vi "MPU6050 Tester.vi"() -> ()   [LabVIEW 2020]
uses:
  Typedefs/LED mode.ctl
  Typedefs/Front Panel Object References.ctl
  Typedefs/GUI Command Cluster.ctl
  Typedefs/GUI Commands.ctl
  Typedefs/SDCP - Standard Message Frame Parameters - FGV - commands.ctl
  Typedefs/SDCP - Serial Port Control - Commands.ctl
  Global Variables/Application Stop.vi
panel:
  in  "Exit Application":bool
  in  "Switch":bool
  in  "Anti clockwise":bool
  in  "Clockwise":bool
  out "Z vibration detected":bool
  out "Y vibration detected":bool
  out "X vibration detected":bool
  out "Z tilt detected":bool
  out "Y tilt detected":bool
  out "X tilt detected":bool
  in  "Save config":bool
  out "Yaw (degrees)":dbl
  out "Pitch (degrees)":dbl
  out "Roll (degrees)":dbl
  in  "Calibrate IMU":bool
  out "IMU orientation":refnum<vi>(3d-picture)
  in  "Serial Port Connect":bool
  in  "Write config":bool
  in  "Read config":bool
  out "Z gyroscope (mDPS)":u16
  out "Y gyroscope (mDPS)":u16
  out "X gyroscope  (mDPS)":u16
  out "Z accelerometer (mG)":u16
  out "Y accelerometer (mG)":u16
  out "X accelerometer (mG)":u16
  out "Z gyroscope raw":u16
  out "Y gyroscope raw":u16
  out "X gyroscope raw":u16
  out "Z accelerometer raw":u16
  out "Y accelerometer raw":u16
  out "X accelerometer raw":u16
  in  "Z LED mode":T1
  in  "Y LED mode":T1
  in  "X LED mode":T1
  in  "Z vib threshold":dbl
  in  "Y vib threshold":dbl
  in  "X vib threshold":dbl
  in  "Z tilt threshold":dbl
  in  "Y tilt threshold":dbl
  in  "X tilt threshold":dbl
  in  "Yaw coefficient":dbl
  in  "Pitch coefficient":dbl
  in  "Roll coefficient":dbl
  in  "Calibration Axis":T2(ring)
  in  "Calibration Points":u8
  in  "Calibration interval (ms)":u8
  in  "Gyroscope full scale value":enum16{"250DPS", "500DPS", "1000DPS", "2000DPS"}(ring)
  in  "Accelerometer full scale value":enum16{"2G", "4G", "8G", "16G"}(ring)
  in  "Baud rate":u32=9600
  in  "COM Port":refnum<visa-resource-name>
  # "IMU Configurations"
  # "Serial Port Configurations"
  # "IMU Raw measurements"
  # "Complementary Filter Configurations"
  # "Tilt Detection Configurations"
  # "IMU Processed measurements"
  # "Vibration Detection Configurations"
  # "LED Configurations"
  # "Screen control"
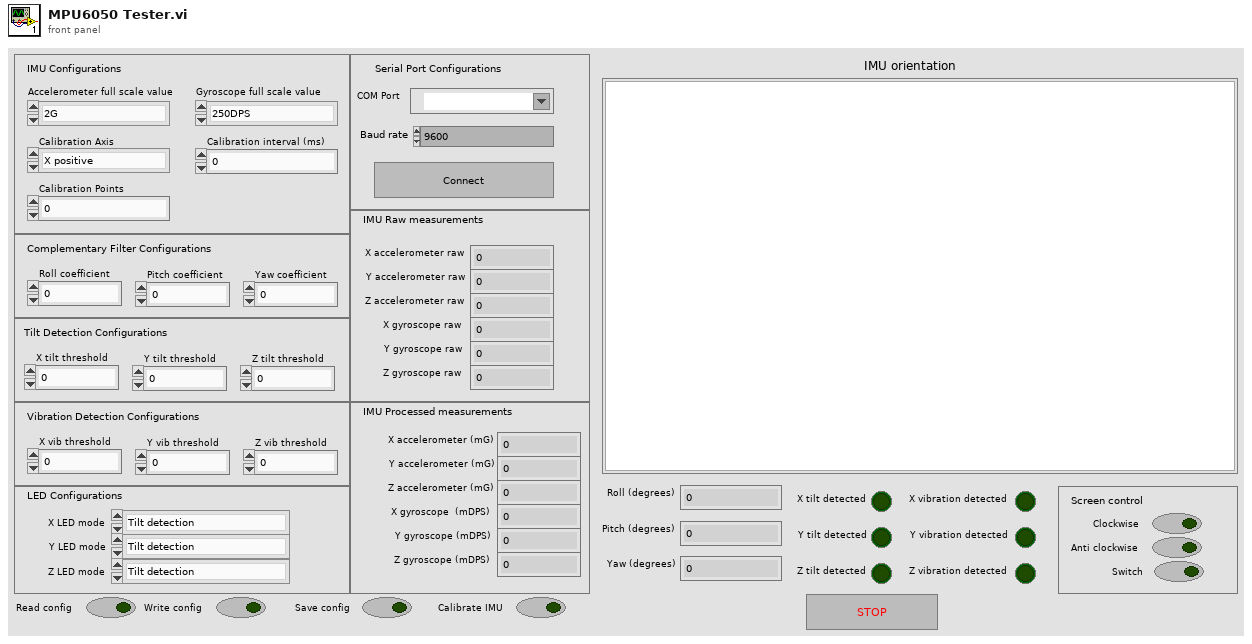
[diagram p1: front panel]
types:
  T1 = typedef "LED mode.ctl" = enum16{"Tilt detection", "Vibration detection", "Accelerometer magnitude", "Gyroscope magnitude", "GPIO test", "PWM test"}
  T2 = enum16{"X positive", "X neagtive", "Y positive", "Y negative", "Z positive", "Z negative"}
  T3 = typedef "SDCP - Standard Message Frame Parameters - FGV - commands.ctl" = enum16{"Write descriptors", "Read descriptors", "Read values", "Load parameters from file", "Write values", "Read all descriptors"}
  T4 = typedef "GUI Command Cluster.ctl" = cluster{"Command":T5, "Data":variant}
  T5 = typedef "GUI Commands.ctl" = enum16{"Serial Port Connect", "Serial Port Disconnect", "Read config", "Write config", "Save config", "Calibrate", "RENC CLK", "RENC ACLK", "RENC SW", "Exit Application"}
  T6 = typedef "Front Panel Object References.ctl" = cluster{"Switch":refnum<vi>, "Anti clockwise":refnum<vi>, "Clockwise":refnum<vi>, "Save config":refnum<vi>, "Calibrate IMU":refnum<vi>, "Serial Port Connect":refnum<vi>, "Write config":refnum<vi>, "Read config":refnum<vi>, "Z LED mode":refnum<vi>, "Y LED mode":refnum<vi>, "X LED mode":refnum<vi>, "Z vib threshold":refnum<vi>, "Y vib threshold":refnum<vi>, "X vib threshold":refnum<vi>, "Z tilt threshold":refnum<vi>, "Y tilt threshold":refnum<vi>, "X tilt threshold":refnum<vi>, "Yaw coefficient":refnum<vi>, "Pitch coefficient":refnum<vi>, "Roll coefficient":refnum<vi>, "Calibration Axis":refnum<vi>, "Calibration Points":refnum<vi>, "Calibration interval (ms)":refnum<vi>, "Gyroscope full scale value":refnum<vi>, "Accelerometer full scale value":refnum<vi>, "Baud rate":refnum<vi>, "COM Port":refnum<vi>, "Z vibration detected":refnum<vi>, "Y vibration detected":refnum<vi>, "X vibration detected":refnum<vi>, "Z tilt detected":refnum<vi>, "Y tilt detected":refnum<vi>, "X tilt detected":refnum<vi>, "Yaw (degrees)":refnum<vi>, "Pitch (degrees)":refnum<vi>, "Roll (degrees)":refnum<vi>, "IMU orientation":refnum<vi>, "Z gyroscope raw (mDPS)":refnum<vi>, "Y gyroscope (mDPS)":refnum<vi>, "X gyroscope raw (mDPS)":refnum<vi>, "Z accelerometer raw (mG)":refnum<vi>, "Y accelerometer raw (mG)":refnum<vi>, "X accelerometer (mG)":refnum<vi>, "Z gyroscope raw":refnum<vi>, "Y gyroscope raw":refnum<vi>, "X gyroscope raw":refnum<vi>, "Z accelerometer raw":refnum<vi>, "Y accelerometer raw":refnum<vi>, "X accelerometer raw":refnum<vi>}
  T7 = typedef "SDCP - SMF parameter descriptors.ctl" = cluster{"Frame name":string, "Frame ID":i32, "Data type":string, "Start Position":i32, "Length":i32, "Factor":dbl, "Offset":dbl, "Parameter name":string, "Value":string}
  T8 = typedef "SDCP - Serial Port Control - Commands.ctl" = enum16{"Open", "Read", "Write", "Get instance", "Close"}
  T9 = enum8{"Enabled", "Disabled", "Disabled and Grayed Out"}
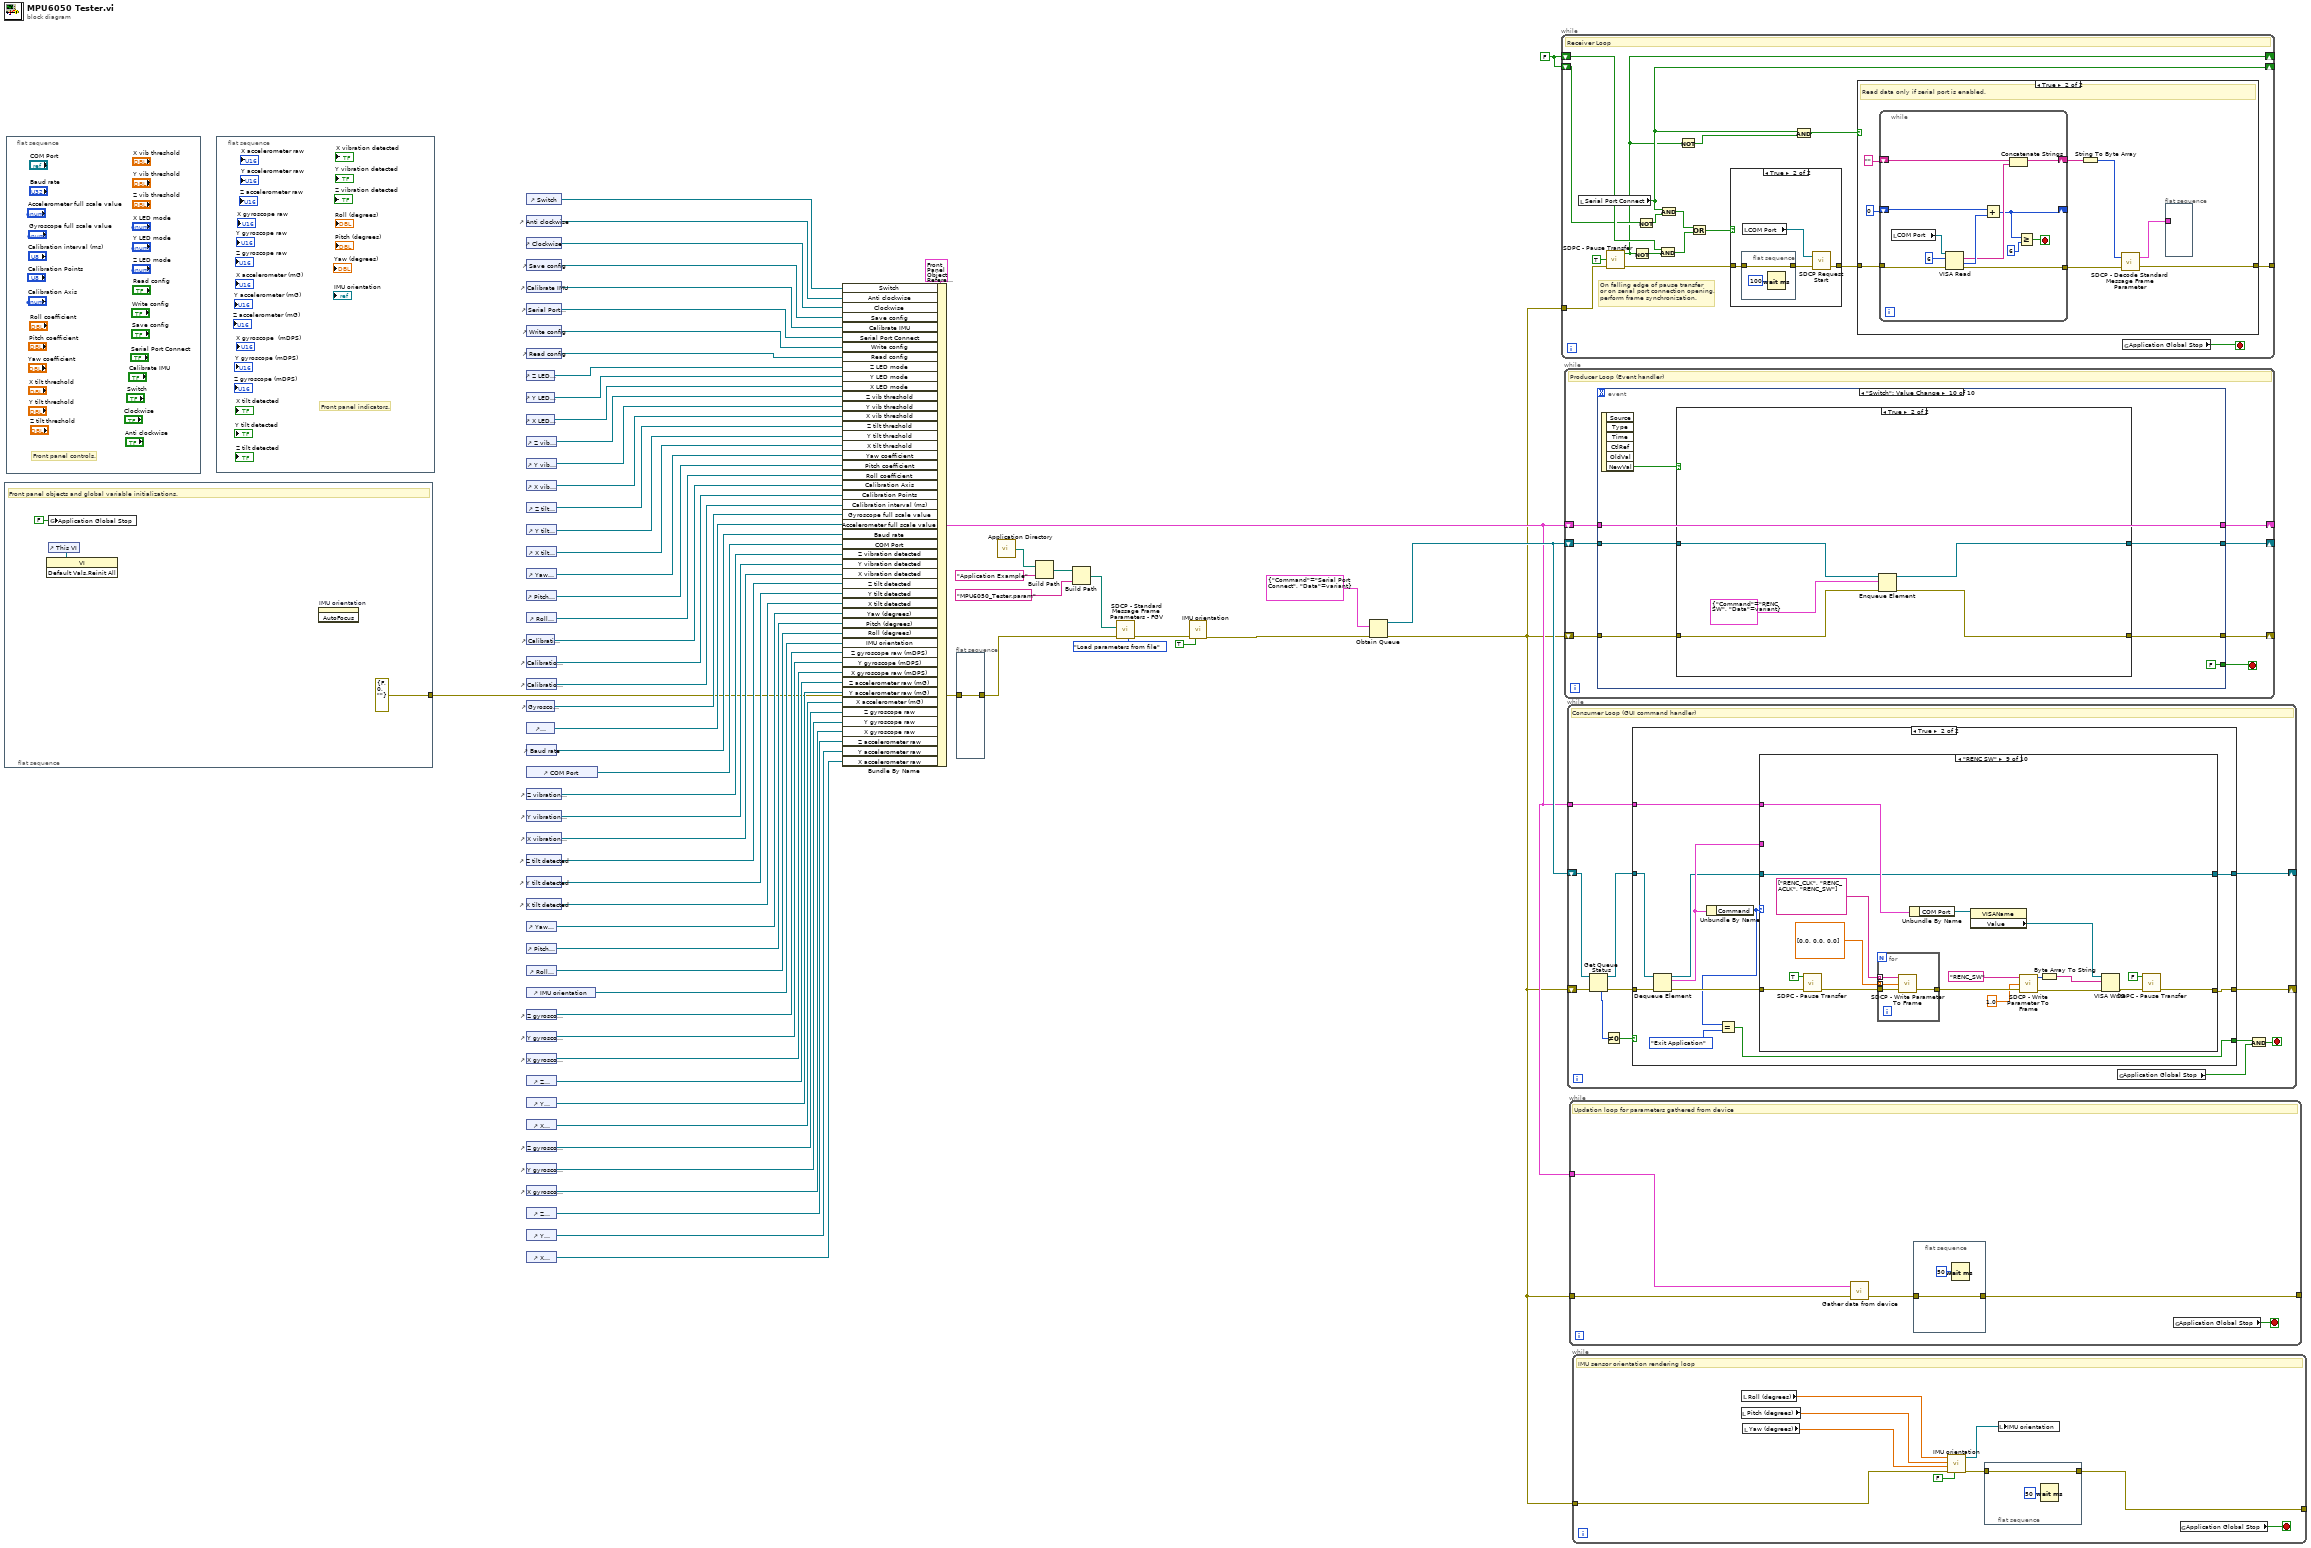
[diagram p0: block diagram]
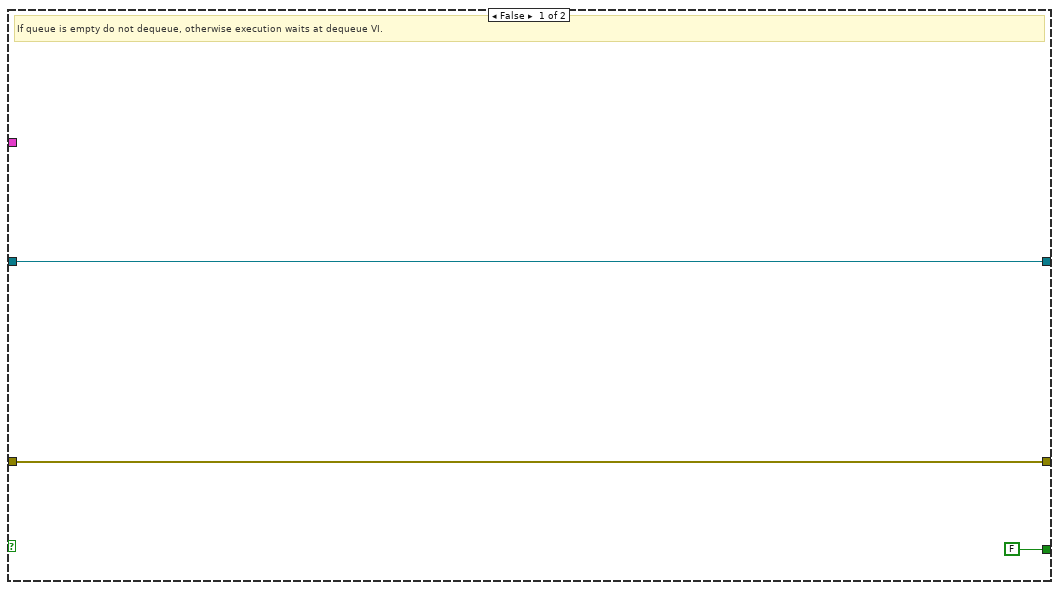
[diagram p4: hidden frame]
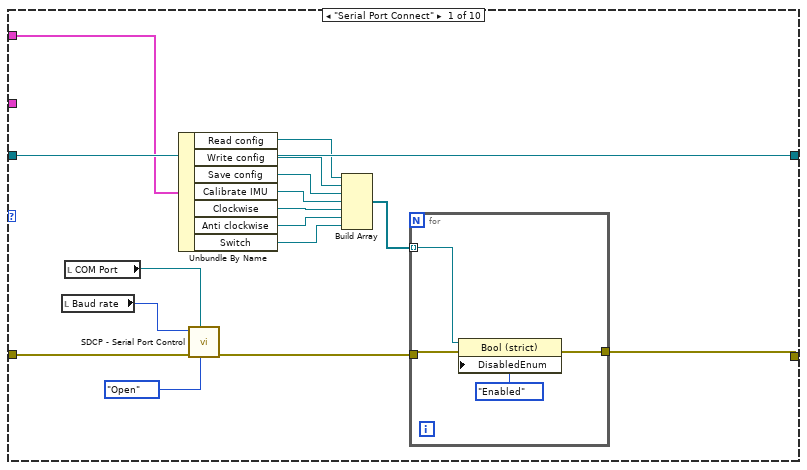
[diagram p5: hidden frame]
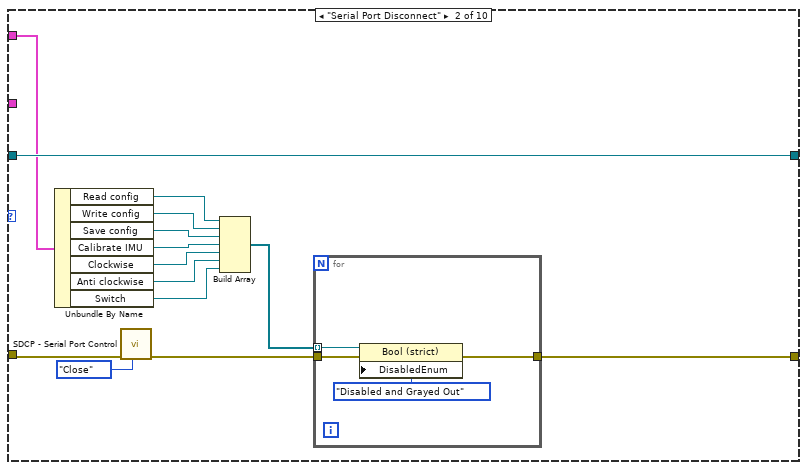
[diagram p6: hidden frame]
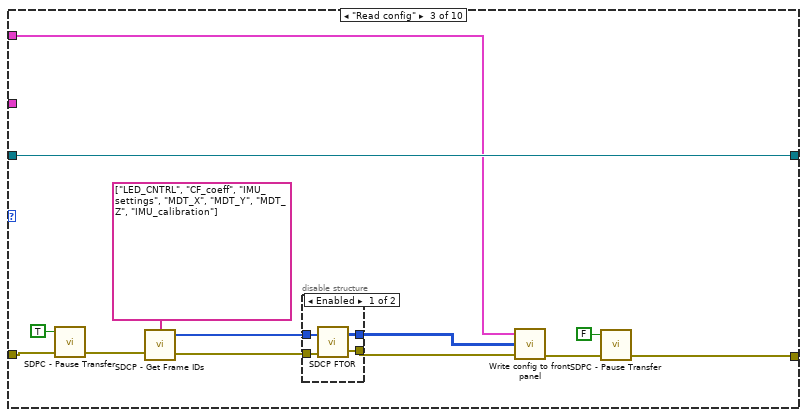
[diagram p7: hidden frame]
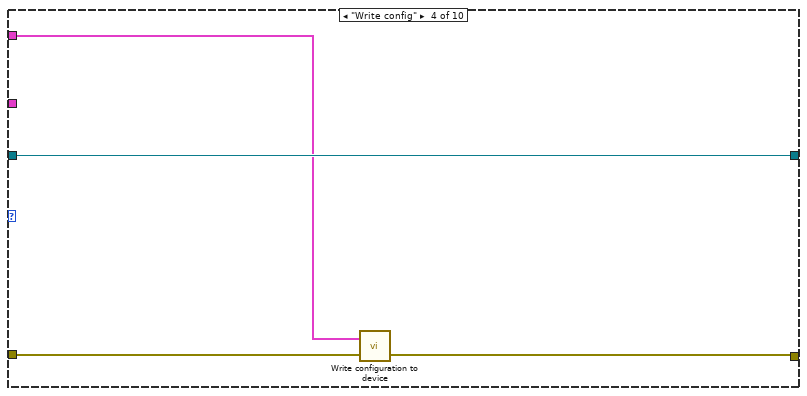
[diagram p9: hidden frame]
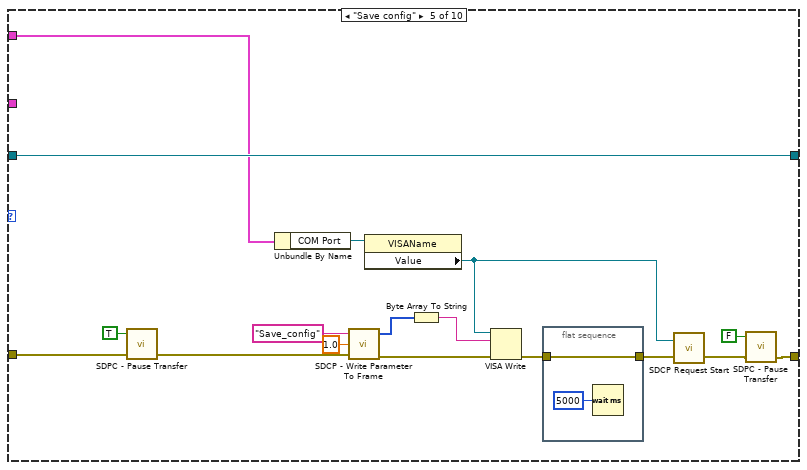
[diagram p10: hidden frame]
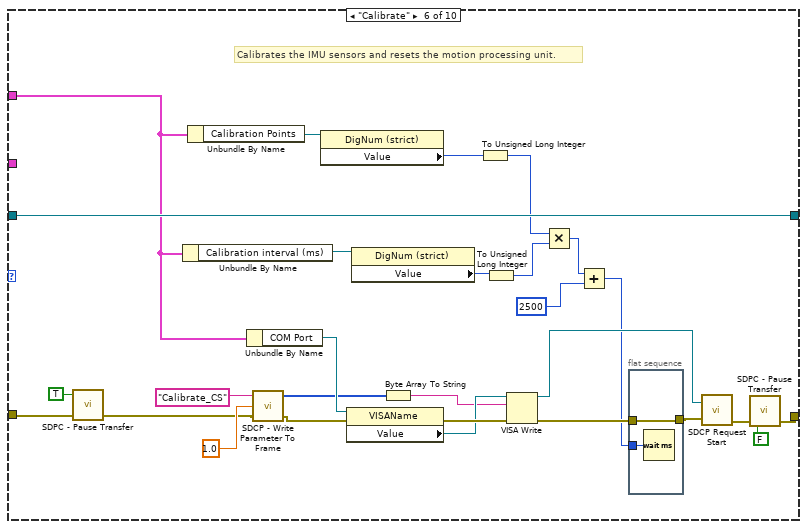
[diagram p11: hidden frame]
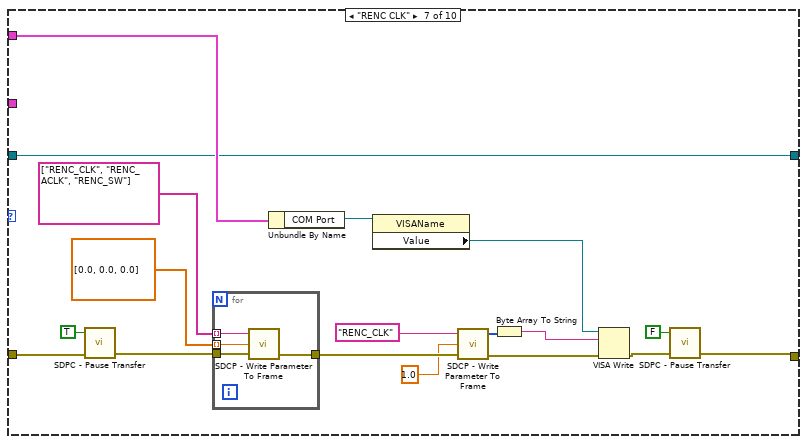
[diagram p12: hidden frame]
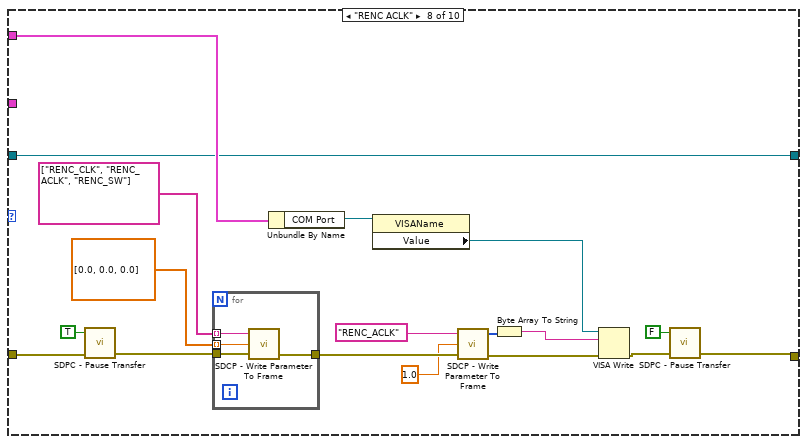
[diagram p13: hidden frame]
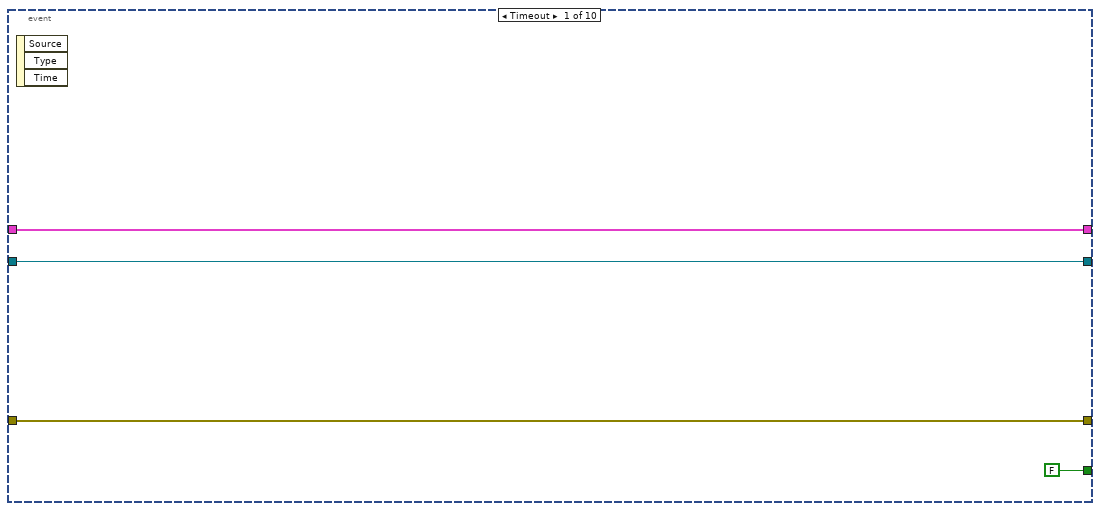
[diagram p15: hidden frame]
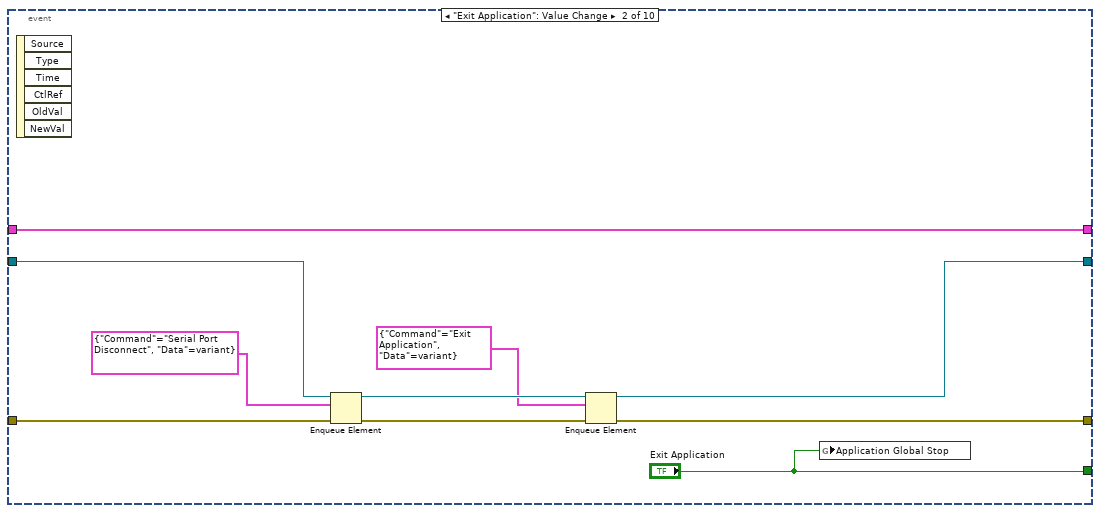
[diagram p16: hidden frame]
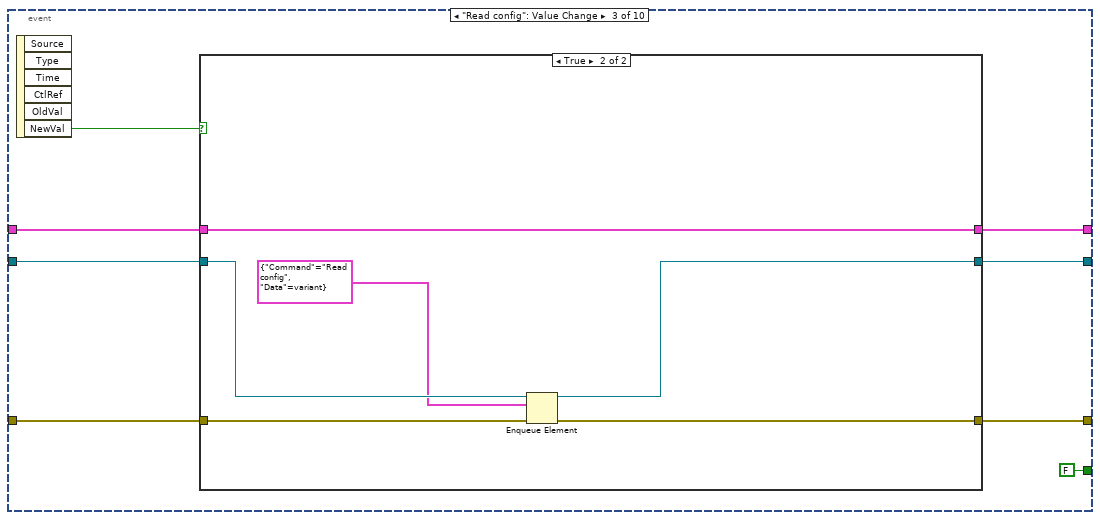
[diagram p17: hidden frame]
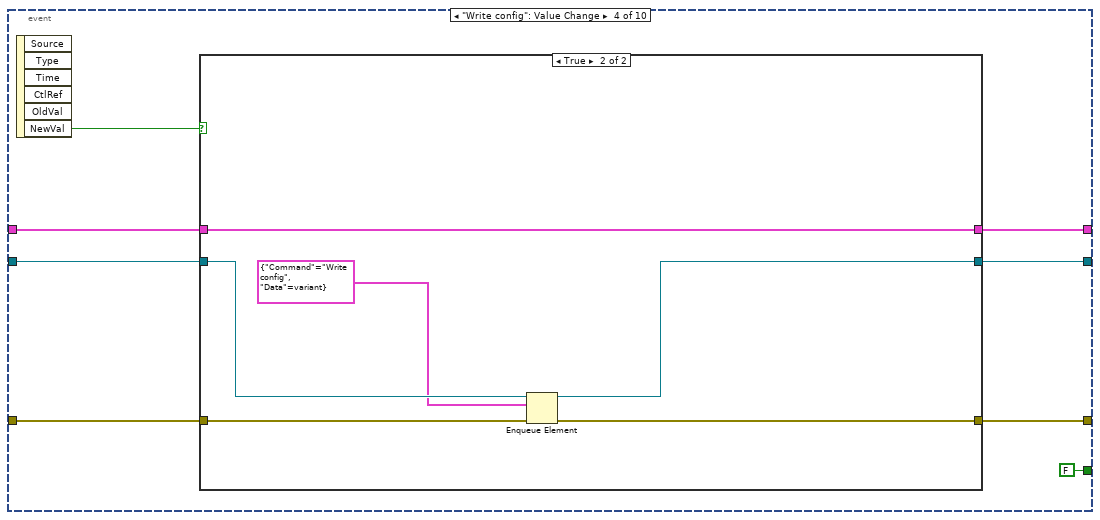
[diagram p19: hidden frame]
diagram:
  w6 = FALSE
  n1 = flat-sequence {
    tunnel: [errorcluster {"status"=FALSE, "code"=0, "source"=""} ("error constant")] -> w15
    frame #0 {
      # "Front panel objects and global variable initializations."
      n2 = global write "Application Stop.vi" "Application Global Stop"(FALSE ("Application Global Stop")) -> ()
      n3 = control-ref of="This VI"() -> (w68:refnum<vi>)
      n4 = invoke class="VI" method="Default Vals.Reinit All"(reference=w68) -> ()  [unwired: 2 in, 3 out]
      n5 = invoke on="IMU orientation" class="SceneGraphDisp (strict)" method="AutoFocus"() -> ()  [unwired: 3 in, 3 out]
    }
  }
  n6 = flat-sequence {
    frame #0 {
      # "Front panel controls."
    }
  }
  n7 = flat-sequence {
    frame #0 {
      # "Front panel indicators."
    }
  }
  n8 = control-ref of="Switch"() -> (w65:refnum<vi>)
  n9 = control-ref of="Anti clockwise"() -> (w64:refnum<vi>)
  n10 = control-ref of="Clockwise"() -> (w63:refnum<vi>)
  n11 = control-ref of="Save config"() -> (w62:refnum<vi>)
  n12 = control-ref of="Calibrate IMU"() -> (w61:refnum<vi>)
  n13 = control-ref of="Serial Port Connect"() -> (w60:refnum<vi>)
  n14 = control-ref of="Write config"() -> (w59:refnum<vi>)
  n15 = control-ref of="Read config"() -> (w58:refnum<vi>)
  n16 = control-ref of="Z LED mode"() -> (w57:refnum<vi>)
  n17 = control-ref of="Y LED mode"() -> (w56:refnum<vi>)
  n18 = control-ref of="X LED mode"() -> (w55:refnum<vi>)
  n19 = control-ref of="Z vib threshold"() -> (w54:refnum<vi>)
  n20 = control-ref of="Y vib threshold"() -> (w53:refnum<vi>)
  n21 = control-ref of="X vib threshold"() -> (w52:refnum<vi>)
  n22 = control-ref of="Z tilt threshold"() -> (w51:refnum<vi>)
  n23 = control-ref of="Y tilt threshold"() -> (w50:refnum<vi>)
  n24 = control-ref of="X tilt threshold"() -> (w49:refnum<vi>)
  n25 = control-ref of="Yaw coefficient"() -> (w48:refnum<vi>)
  n26 = control-ref of="Pitch coefficient"() -> (w47:refnum<vi>)
  n27 = control-ref of="Roll coefficient"() -> (w46:refnum<vi>)
  n28 = control-ref of="Calibration Axis"() -> (w45:refnum<vi>)
  n29 = control-ref of="Calibration Points"() -> (w44:refnum<vi>)
  n30 = control-ref of="Calibration interval (ms)"() -> (w43:refnum<vi>)
  n31 = control-ref of="Gyroscope full scale value"() -> (w42:refnum<vi>)
  n32 = control-ref of="Accelerometer full scale value"() -> (w41:refnum<vi>)
  n33 = control-ref of="Baud rate"() -> (w40:refnum<vi>)
  n34 = control-ref of="COM Port"() -> (w39:refnum<vi>)
  n35 = control-ref of="Z vibration detected"() -> (w38:refnum<vi>)
  n36 = control-ref of="Y vibration detected"() -> (w37:refnum<vi>)
  n37 = control-ref of="X vibration detected"() -> (w36:refnum<vi>)
  n38 = control-ref of="Z tilt detected"() -> (w35:refnum<vi>)
  n39 = control-ref of="Y tilt detected"() -> (w34:refnum<vi>)
  n40 = control-ref of="X tilt detected"() -> (w33:refnum<vi>)
  n41 = control-ref of="Yaw (degrees)"() -> (w32:refnum<vi>)
  n42 = control-ref of="Pitch (degrees)"() -> (w31:refnum<vi>)
  n43 = control-ref of="Roll (degrees)"() -> (w30:refnum<vi>)
  n44 = control-ref of="IMU orientation"() -> (w29:refnum<vi>)
  n45 = control-ref of="Z gyroscope (mDPS)"() -> (w28:refnum<vi>)
  n46 = control-ref of="Y gyroscope (mDPS)"() -> (w27:refnum<vi>)
  n47 = control-ref of="X gyroscope  (mDPS)"() -> (w26:refnum<vi>)
  n48 = control-ref of="Z accelerometer (mG)"() -> (w25:refnum<vi>)
  n49 = control-ref of="Y accelerometer (mG)"() -> (w24:refnum<vi>)
  n50 = control-ref of="X accelerometer (mG)"() -> (w23:refnum<vi>)
  n51 = control-ref of="Z gyroscope raw"() -> (w22:refnum<vi>)
  n52 = control-ref of="Y gyroscope raw"() -> (w21:refnum<vi>)
  n53 = control-ref of="X gyroscope raw"() -> (w20:refnum<vi>)
  n54 = control-ref of="Z accelerometer raw"() -> (w19:refnum<vi>)
  n55 = control-ref of="Y accelerometer raw"() -> (w18:refnum<vi>)
  n56 = control-ref of="X accelerometer raw"() -> (w17:refnum<vi>)
  n57 = Bundle By Name(cluster=T6 {"Switch"=refnum, "Anti clockwise"=refnum, "Clockwise"=refnum, "Save config"=refnum, "Calibrate IMU"=refnum, "Serial Port Connect"=refnum, "Write config"=refnum, "Read config"=refnum, "Z LED mode"=refnum, "Y LED mode"=refnum, "X LED mode"=refnum, "Z vib threshold"=refnum, "Y vib threshold"=refnum, "X vib threshold"=refnum, "Z tilt threshold"=refnum, "Y tilt threshold"=refnum, "X tilt threshold"=refnum, "Yaw coefficient"=refnum, "Pitch coefficient"=refnum, "Roll coefficient"=refnum, "Calibration Axis"=refnum, "Calibration Points"=refnum, "Calibration interval (ms)"=refnum, "Gyroscope full scale value"=refnum, "Accelerometer full scale value"=refnum, "Baud rate"=refnum, "COM Port"=refnum, "Z vibration detected"=refnum, "Y vibration detected"=refnum, "X vibration detected"=refnum, "Z tilt detected"=refnum, "Y tilt detected"=refnum, "X tilt detected"=refnum, "Yaw (degrees)"=refnum, "Pitch (degrees)"=refnum, "Roll (degrees)"=refnum, "IMU orientation"=refnum, "Z gyroscope raw (mDPS)"=refnum, "Y gyroscope (mDPS)"=refnum, "X gyroscope raw (mDPS)"=refnum, "Z accelerometer raw (mG)"=refnum, "Y accelerometer raw (mG)"=refnum, "X accelerometer (mG)"=refnum, "Z gyroscope raw"=refnum, "Y gyroscope raw"=refnum, "X gyroscope raw"=refnum, "Z accelerometer raw"=refnum, "Y accelerometer raw"=refnum, "X accelerometer raw"=refnum} ("Front Panel Object References"), "Switch"=w65, "Anti clockwise"=w64, "Clockwise"=w63, "Save config"=w62, "Calibrate IMU"=w61, "Serial Port Connect"=w60, "Write config"=w59, "Read config"=w58, "Z LED mode"=w57, "Y LED mode"=w56, "X LED mode"=w55, "Z vib threshold"=w54, "Y vib threshold"=w53, "X vib threshold"=w52, "Z tilt threshold"=w51, "Y tilt threshold"=w50, "X tilt threshold"=w49, "Yaw coefficient"=w48, "Pitch coefficient"=w47, "Roll coefficient"=w46, "Calibration Axis"=w45, "Calibration Points"=w44, "Calibration interval (ms)"=w43, "Gyroscope full scale value"=w42, "Accelerometer full scale value"=w41, "Baud rate"=w40, "COM Port"=w39, "Z vibration detected"=w38, "Y vibration detected"=w37, "X vibration detected"=w36, "Z tilt detected"=w35, "Y tilt detected"=w34, "X tilt detected"=w33, "Yaw (degrees)"=w32, "Pitch (degrees)"=w31, "Roll (degrees)"=w30, "IMU orientation"=w29, "Z gyroscope raw (mDPS)"=w28, "Y gyroscope (mDPS)"=w27, "X gyroscope raw (mDPS)"=w26, "Z accelerometer raw (mG)"=w25, "Y accelerometer raw (mG)"=w24, "X accelerometer (mG)"=w23, "Z gyroscope raw"=w22, "Y gyroscope raw"=w21, "X gyroscope raw"=w20, "Z accelerometer raw"=w19, "Y accelerometer raw"=w18, "X accelerometer raw"=w17) -> (w5:T6)
  n58 = flat-sequence {
    tunnel: w15 -> [w70]
    tunnel: [w70] -> w13
    frame #0 {
    }
  }
  n59 = call <vilib>:"Application Directory.vi"() -> ("Application Directory"=w11:path)
  n60 = Build Path(base path=w11, name or relative path="Application Example") -> (appended path=w9:path)
  n61 = Build Path(base path=w9, name or relative path="MPU6050_Tester.param") -> (appended path=w7:path)
  n62 = call "SDCP - Standard Message Frame Parameters - FGV.vi"("Parameter file path"=w7, "error in (no error)"=w13, "Command"=SDCP_-_Standard_Message_Frame_Parameters_-_FGV_-_commands."Load parameters from file") -> ("error out"=w3:errorcluster)  [unwired: 4 in, 1 out]
  n63 = call "IMU orientation.vi"("Initialize ?"=TRUE, "error in (no error)"=w3) -> ("error out"=w2:errorcluster)  [unwired: 8 in, 1 out]
  n64 = Obtain Queue(element data type=T4 {"Command"=enum."Serial Port Connect", "Data"=variant}, error in (no error)=w2) -> (queue out=w14:refnum<queue>, error out=w4:errorcluster)  [unwired: 3 in, 1 out]
  n65 = while {
    tunnel: w4 -> [w85]
    shift-right: [w71] -> _
    shift-left: w6 -> [w83]
    shift-right: [w73] -> _
    shift-left: w6 -> [w81]
    tunnel: [w75] -> _
    stop <- w87 stop-if-true
    # "On falling edge of pause transfer\nor on serial port connection opening,\nperform frame synchronization."
    # "Receiver Loop"
    n66 = local read "Serial Port Connect"() -> (w73:bool)
    n67 = call "SDPC - Pause Transfer.vi"("error in (no error)"=w85, "RD/nWR"=TRUE) -> ("error out"=w77:errorcluster, "Transfer paused"=w71:bool)  [unwired: 2 in]
    n68 = Not(x=w71) -> (.not. x?=w84:bool)
    n69 = Not(x=w81) -> (.not. x?=w82:bool)
    n70 = And(x=w83, y=w84) -> (x .and. y?=w79:bool)
    n71 = And(x=w73, y=w82) -> (x .and. y?=w80:bool)
    n72 = Not(x=w71) -> (.not. x?=w72:bool)
    n73 = Or(x=w80, y=w79) -> (x .or. y?=w78:bool)
    n74 = case shown="True" w78 {
      tunnel: w77 -> [w109 w111]
      tunnel: [w109 w113] -> w76
      frame False {
      }
      frame True {
        n75 = flat-sequence {
          tunnel: w111 -> [w115]
          tunnel: [w115] -> w110
          frame #0 {
            n76 = Wait (ms)(milliseconds to wait=u32 100) -> ()  [unwired: 1 out]
          }
        }
        n77 = local read "COM Port"() -> (w112:refnum<visa-resource-name>)
        n78 = call "SDCP Request Start.vi"("error in (no error)"=w110, "COM Port"=w112) -> ("error out"=w113:errorcluster)  [unwired: 1 out]
      }
    }
    n79 = And(x=w73, y=w72) -> (x .and. y?=w74:bool)
    n80 = case shown="True" w74 {
      tunnel: w76 -> [w88 w96]
      tunnel: [w88 w90] -> w75
      frame False {
      }
      frame True {
        # "Read data only if serial port is enabled."
        n81 = while {
          tunnel: w96 -> [w108]
          shift-right: [w100] -> _
          shift-left: 0 -> [w106]
          shift-right: [w101] -> w93
          shift-left: "" -> [w103]
          tunnel: [w97] -> w92
          stop <- w98 stop-if-true
          n82 = local read "COM Port"() -> (w107:refnum<visa-resource-name>)
          n83 = VISA Read(VISA resource name=w107, byte count=u32 6, error in (no error)=w108) -> (read buffer=w102:string, return count=w104:u32, error out=w97:errorcluster)  [unwired: 1 out]
          n84 = Add(x=w106, y=w104) -> (x+y=w100:u32)
          n85 = Concatenate Strings(w103, w102) -> (w101:string)
          n86 = Greater Or Equal?(x=w100, y=u32 6) -> (x >= y?=w98:bool)
        }
        n87 = String To Byte Array(string=w93) -> (unsigned byte array=w91:u8[])
        n88 = call "SDCP - Decode Standard Message Frame Parameter.vi"("error in (no error)"=w92, "Bytes in"=w91) -> ("error out"=w90:errorcluster, "SMF Parameters out"=w89:T7[])
        n89 = flat-sequence {
          tunnel: w89 -> [_]
          frame #0 {
          }
        }
      }
    }
    n90 = global read "Application Stop.vi" "Application Global Stop"() -> (w87:bool)
  }
  n91 = while {
    shift-right: [w118] -> _
    shift-left: w5 -> [w122]
    shift-right: [w120] -> _
    shift-left: w4 -> [w121]
    shift-right: [w116] -> _
    shift-left: w14 -> [w117]
    stop <- w119 stop-if-true
    # "Producer Loop (Event handler)"
    n92 = event shown="[9] \"Switch\": Value Change" {
      selector: _ -> [_ _ _ _ _ _ _ _ _ _]
      dyn-events: _ -> [_ _ _ _ _ _ _ _ _ _]
      timeout: _ -> [_ _ _ _ _ _ _ _ _ _]
      tunnel: w122 -> [w124 w136 w138 w155 w172 w191 w210 w227 w241 w255]
      tunnel: w121 -> [w126 w134 w142 w159 w176 w193 w214 w230 w244 w258]
      tunnel: [w126 w128 w141 w158 w175 w189 w208 w228 w242 w256] -> w120
      tunnel: [FALSE "Exit Application" FALSE ("Exit Application") FALSE ("Exit Application") FALSE ("Exit Application") FALSE ("Exit Application") FALSE ("Exit Application") FALSE ("Exit Application") FALSE ("Exit Application") FALSE ("Exit Application")] -> w119
      tunnel: [w124 w136 w137 w154 w171 w190 w209 w227 w241 w255] -> w118
      tunnel: w117 -> [w123 w133 w140 w157 w174 w192 w212 w226 w240 w254]
      tunnel: [w123 w127 w139 w156 w173 w188 w211 w225 w239 w253] -> w116
      event Timeout {
        n93 = event-data() -> ()  [unwired: 1 in, 3 out]
      }
      event "Exit Application": Value Change {
        n94 = event-data() -> ()  [unwired: 1 in, 6 out]
        n95 = Enqueue Element(queue=w133, element=T4 {"Command"=enum."Serial Port Disconnect", "Data"=variant}, error in (no error)=w134) -> (queue out=w130:refnum<queue>, error out=w131:errorcluster)  [unwired: 1 in, 1 out]
        n96 = Enqueue Element(queue=w130, element=T4 {"Command"=enum."Exit Application", "Data"=variant}, error in (no error)=w131) -> (queue out=w127:refnum<queue>, error out=w128:errorcluster)  [unwired: 1 in, 1 out]
        n97 = global write "Application Stop.vi" "Application Global Stop"("Exit Application") -> ()
      }
      event "Read config": Value Change {
        n98 = event-data() -> ("NewVal"=w143:bool)  [unwired: 1 in, 5 out]
        n99 = case shown="True" w143 {
          tunnel: w142 -> [w147 w152]
          tunnel: [w147 w149] -> w141
          tunnel: w140 -> [w146 w151]
          tunnel: [w146 w150] -> w139
          tunnel: w138 -> [w145 w153]
          tunnel: [w145 w153] -> w137
          frame False {
          }
          frame True {
            n100 = Enqueue Element(queue=w151, element=T4 {"Command"=enum."Read config", "Data"=variant}, error in (no error)=w152) -> (queue out=w150:refnum<queue>, error out=w149:errorcluster)  [unwired: 1 in, 1 out]
          }
        }
      }
      event "Write config": Value Change {
        n101 = event-data() -> ("NewVal"=w160:bool)  [unwired: 1 in, 5 out]
        n102 = case shown="True" w160 {
          tunnel: w159 -> [w164 w169]
          tunnel: [w164 w166] -> w158
          tunnel: w157 -> [w163 w168]
          tunnel: [w163 w167] -> w156
          tunnel: w155 -> [w162 w170]
          tunnel: [w162 w170] -> w154
          frame False {
          }
          frame True {
            n103 = Enqueue Element(queue=w168, element=T4 {"Command"=enum."Write config", "Data"=variant}, error in (no error)=w169) -> (queue out=w167:refnum<queue>, error out=w166:errorcluster)  [unwired: 1 in, 1 out]
          }
        }
      }
      event "Save config": Value Change {
        n104 = event-data() -> ("NewVal"=w177:bool)  [unwired: 1 in, 5 out]
        n105 = case shown="True" w177 {
          tunnel: w176 -> [w181 w186]
          tunnel: [w181 w183] -> w175
          tunnel: w174 -> [w180 w185]
          tunnel: [w180 w184] -> w173
          tunnel: w172 -> [w179 w187]
          tunnel: [w179 w187] -> w171
          frame False {
          }
          frame True {
            n106 = Enqueue Element(queue=w185, element=T4 {"Command"=enum."Save config", "Data"=variant}, error in (no error)=w186) -> (queue out=w184:refnum<queue>, error out=w183:errorcluster)  [unwired: 1 in, 1 out]
          }
        }
      }
      event "Serial Port Connect": Value Change {
        n107 = event-data() -> ("NewVal"=w194:bool)  [unwired: 1 in, 5 out]
        n108 = case shown="False" w194 {
          tunnel: w193 -> [w201 w207]
          tunnel: w192 -> [w200 w206]
          tunnel: w191 -> [w199 w205]
          tunnel: [w199 w205] -> w190
          tunnel: [w197 w203] -> w189
          tunnel: [w196 w202] -> w188
          frame True {
            n109 = Enqueue Element(queue=w200, element=T4 {"Command"=enum."Serial Port Connect", "Data"=variant}, error in (no error)=w201) -> (queue out=w196:refnum<queue>, error out=w197:errorcluster)  [unwired: 1 in, 1 out]
          }
          frame False {
            n110 = Enqueue Element(queue=w206, element=T4 {"Command"=enum."Serial Port Disconnect", "Data"=variant}, error in (no error)=w207) -> (queue out=w202:refnum<queue>, error out=w203:errorcluster)  [unwired: 1 in, 1 out]
          }
        }
      }
      event "Calibrate IMU": Value Change {
        n111 = event-data() -> ("NewVal"=w213:bool)  [unwired: 1 in, 5 out]
        n112 = case shown="True" w213 {
          tunnel: w214 -> [w216 w224]
          tunnel: w212 -> [w218 w223]
          tunnel: [w218 w221] -> w211
          tunnel: w210 -> [w217 w220]
          tunnel: [w217 w220] -> w209
          tunnel: [w216 w219] -> w208
          frame False {
          }
          frame True {
            n113 = Enqueue Element(queue=w223, element=T4 {"Command"=enum."Calibrate", "Data"=variant}, error in (no error)=w224) -> (queue out=w221:refnum<queue>, error out=w219:errorcluster)  [unwired: 1 in, 1 out]
          }
        }
      }
      event "Clockwise": Value Change {
        n114 = event-data() -> ("NewVal"=w229:bool)  [unwired: 1 in, 5 out]
        n115 = case shown="True" w229 {
          tunnel: w230 -> [w233 w238]
          tunnel: [w233 w237] -> w228
          tunnel: w226 -> [w232 w236]
          tunnel: [w232 w234] -> w225
          frame False {
          }
          frame True {
            n116 = Enqueue Element(queue=w236, element=T4 {"Command"=enum."RENC CLK", "Data"=variant}, error in (no error)=w238) -> (queue out=w234:refnum<queue>, error out=w237:errorcluster)  [unwired: 1 in, 1 out]
          }
        }
      }
      event "Anti clockwise": Value Change {
        n117 = event-data() -> ("NewVal"=w243:bool)  [unwired: 1 in, 5 out]
        n118 = case shown="True" w243 {
          tunnel: w244 -> [w247 w252]
          tunnel: [w247 w251] -> w242
          tunnel: w240 -> [w246 w250]
          tunnel: [w246 w248] -> w239
          frame False {
          }
          frame True {
            n119 = Enqueue Element(queue=w250, element=T4 {"Command"=enum."RENC ACLK", "Data"=variant}, error in (no error)=w252) -> (queue out=w248:refnum<queue>, error out=w251:errorcluster)  [unwired: 1 in, 1 out]
          }
        }
      }
      event "Switch": Value Change {
        n120 = event-data() -> ("NewVal"=w257:bool)  [unwired: 1 in, 5 out]
        n121 = case shown="True" w257 {
          tunnel: w258 -> [w261 w266]
          tunnel: [w261 w265] -> w256
          tunnel: w254 -> [w260 w264]
          tunnel: [w260 w262] -> w253
          frame False {
          }
          frame True {
            n122 = Enqueue Element(queue=w264, element=T4 {"Command"=enum."RENC SW", "Data"=variant}, error in (no error)=w266) -> (queue out=w262:refnum<queue>, error out=w265:errorcluster)  [unwired: 1 in, 1 out]
          }
        }
      }
    }
  }
  n123 = while {
    shift-right: [w271] -> _
    shift-left: w14 -> [w277]
    shift-right: [w273] -> _
    shift-left: w4 -> [w278]
    tunnel: w5 -> [w270]
    stop <- w269 stop-if-true
    # "Consumer Loop (GUI command handler)"
    n124 = Get Queue Status(queue=w277, error in (no error)=w278) -> (queue out=w272:refnum<queue>, error out=w274:errorcluster, # elements in queue=w276:i32)  [unwired: 1 in, 5 out]
    n125 = Not Equal To 0?(x=w276) -> (x != 0?=w275:bool)
    n126 = case shown="True" w275 {
      tunnel: w274 -> [w281 w292]
      tunnel: [w281 w288] -> w273
      tunnel: w272 -> [w280 w291]
      tunnel: [w280 w286] -> w271
      tunnel: w270 -> [_ w285]
      tunnel: [FALSE w282] -> w267
      frame False {
        # "If queue is empty do not dequeue, otherwise execution waits at dequeue VI."
      }
      frame True {
        n127 = Dequeue Element(queue=w291, error in (no error)=w292) -> (queue out=w287:refnum<queue>, element=w289:T4, error out=w290:errorcluster)  [unwired: 1 in, 1 out]
        n128 = Unbundle By Name(w289) -> ("Command"=w284:T5)
        n129 = Equal?(x=w284, y=GUI_Commands."Exit Application") -> (x = y?=w282:bool)
        n130 = case shown="\"RENC SW\"" w284 {
          tunnel: w290 -> [w308 w325 w336 w351 w361 w377 w419 w441 w463 w469]
          tunnel: w289 -> [_ _ _ _ _ _ _ _ _ _]
          tunnel: [w293 w313 w332 w349 w358 w373 w404 w426 w448 w469] -> w288
          tunnel: w287 -> [w304 w326 w343 w352 w369 w399 w402 w424 w446 w468]
          tunnel: [w304 w326 w343 w352 w369 w399 w402 w424 w446 w468] -> w286
          tunnel: w285 -> [w303 w323 w337 w350 w365 w386 w411 w433 w455 _]
          frame "Serial Port Connect" {
            n131 = local read "Baud rate"() -> (w306:u32)
            n132 = local read "COM Port"() -> (w307:refnum<visa-resource-name>)
            n133 = Unbundle By Name(w303) -> ("Read config"=w302:refnum<vi>, "Write config"=w301:refnum<vi>, "Save config"=w300:refnum<vi>, "Calibrate IMU"=w299:refnum<vi>, "Clockwise"=w298:refnum<vi>, "Anti clockwise"=w297:refnum<vi>, "Switch"=w296:refnum<vi>)
            n134 = call "SDCP - Serial Port Control.vi"("Command"=SDCP_-_Serial_Port_Control_-_Commands."Open", "VISA resource name"=w307, "error in (no error)"=w308, "Baud rate"=w306) -> ("error out"=w294:errorcluster)  [unwired: 4 in, 3 out]
            n135 = Build Array(w302, w301, w300, w299, w298, w297, w296) -> (w295:refnum<vi>[])
            n136 = for {
              tunnel: w295 -> [w311] mode=indexing
              tunnel: w294 -> [w312]
              tunnel: [w309] -> w293
              n137 = property class="Bool (strict)"(reference=w311, error in=w312, "DisabledEnum"=T9."Enabled" ("Disabled")) -> (error out=w309:errorcluster)  [unwired: 1 out]
            }
          }
          frame "Serial Port Disconnect" {
            n138 = Unbundle By Name(w323) -> ("Read config"=w322:refnum<vi>, "Write config"=w321:refnum<vi>, "Save config"=w320:refnum<vi>, "Calibrate IMU"=w319:refnum<vi>, "Clockwise"=w318:refnum<vi>, "Anti clockwise"=w317:refnum<vi>, "Switch"=w316:refnum<vi>)
            n139 = call "SDCP - Serial Port Control.vi"("Command"=SDCP_-_Serial_Port_Control_-_Commands."Close", "error in (no error)"=w325) -> ("error out"=w315:errorcluster)  [unwired: 6 in, 3 out]
            n140 = Build Array(w322, w321, w320, w319, w318, w317, w316) -> (w314:refnum<vi>[])
            n141 = for {
              tunnel: w315 -> [w330]
              tunnel: w314 -> [w329] mode=indexing
              tunnel: [w327] -> w313
              n142 = property class="Bool (strict)"(reference=w329, error in=w330, "DisabledEnum"=T9."Disabled and Grayed Out" ("Disabled")) -> (error out=w327:errorcluster)  [unwired: 1 out]
            }
          }
          frame "Read config" {
            n143 = call "SDPC - Pause Transfer.vi"("error in (no error)"=w336, "Pause transfer"=TRUE) -> ("error out"=w334:errorcluster)  [unwired: 2 in, 1 out]
            n144 = call "SDCP - Get Frame IDs.vi"("error in (no error)"=w334, "Frame names"=string[] ["LED_CNTRL", "CF_coeff", "IMU_settings", "MDT_X", "MDT_Y", "MDT_Z", "IMU_calibration"]) -> ("error out"=w341:errorcluster, "Frame IDs"=w340:u8[])
            n145 = disable-structure shown="Enabled" {
              disable-tunnel: w341 -> [w347 w348]
              disable-tunnel: w340 -> [w346 _]
              disable-tunnel: [w345 w348] -> w339
              disable-tunnel: [w344 _] -> w338
              frame Enabled {
                n146 = call "SDCP FTOR.vi"("error in (no error)"=w347, "FID"=w346) -> ("error out"=w345:errorcluster, "Received frames"=w344:u8[][])
              }
              frame Disabled {
              }
            }
            n147 = call "Write config to front panel.vi"("error in (no error)"=w339, "frames in"=w338, "FP ref in"=w337) -> ("error out"=w333:errorcluster)  [unwired: 2 in]
            n148 = call "SDPC - Pause Transfer.vi"("error in (no error)"=w333, "Pause transfer"=FALSE) -> ("error out"=w332:errorcluster)  [unwired: 2 in, 1 out]
          }
          frame "Write config" {
            n149 = call "Write configuration to device.vi"("error in (no error)"=w351, "FP ref in"=w350) -> ("error out"=w349:errorcluster)  [unwired: 1 in]
          }
          frame "Save config" {
            n150 = call "SDPC - Pause Transfer.vi"("error in (no error)"=w361, "Pause transfer"=TRUE) -> ("error out"=w359:errorcluster)  [unwired: 2 in, 1 out]
            n151 = Unbundle By Name(w365) -> ("COM Port"=w364:refnum<vi>)
            n152 = call "SDCP - Write Parameter To Frame.vi"("error in (no error)"=w359, "Value"=1.0, "Parameter Name"="Save_config") -> ("error out"=w366:errorcluster, "Encoded message frame"=w363:u8[])  [unwired: 1 in]
            n153 = property class="VISAName"(reference=w364) -> ("Value"=w353:refnum<visa-resource-name>)  [unwired: 1 in, 2 out]
            n154 = Byte Array To String(unsigned byte array=w363) -> (string=w362:string)
            n155 = VISA Write(VISA resource name=w353, write buffer=w362, error in (no error)=w366) -> (error out=w356:errorcluster)  [unwired: 2 out]
            n156 = flat-sequence {
              tunnel: w356 -> [w371]
              tunnel: [w371] -> w355
              frame #0 {
                n157 = Wait (ms)(milliseconds to wait=u32 5000) -> ()  [unwired: 1 out]
              }
            }
            n158 = call "SDCP Request Start.vi"("error in (no error)"=w355, "COM Port"=w353) -> ("error out"=w354:errorcluster)  [unwired: 1 out]
            n159 = call "SDPC - Pause Transfer.vi"("error in (no error)"=w354, "Pause transfer"=FALSE) -> ("error out"=w358:errorcluster)  [unwired: 2 in, 1 out]
          }
          frame "Calibrate" {
            # "Calibrates the IMU sensors and resets the motion processing unit."
            n160 = call "SDPC - Pause Transfer.vi"("error in (no error)"=w377, "Pause transfer"=TRUE) -> ("error out"=w376:errorcluster)  [unwired: 2 in, 1 out]
            n161 = Unbundle By Name(w386) -> ("Calibration interval (ms)"=w385:refnum<vi>)
            n162 = Unbundle By Name(w386) -> ("Calibration Points"=w387:refnum<vi>)
            n163 = Unbundle By Name(w386) -> ("COM Port"=w395:refnum<vi>)
            n164 = call "SDCP - Write Parameter To Frame.vi"("error in (no error)"=w376, "Value"=1.0, "Parameter Name"="Calibrate_CS") -> ("error out"=w396:errorcluster, "Encoded message frame"=w392:u8[])  [unwired: 1 in]
            n165 = property class="DigNum (strict)"(reference=w387) -> ("Value"=w384:u8)  [unwired: 1 in, 2 out]
            n166 = property class="VISAName"(reference=w395, error in=w396) -> (error out=w394:errorcluster, "Value"=w393:refnum<visa-resource-name>)  [unwired: 1 out]
            n167 = property class="DigNum (strict)"(reference=w385) -> ("Value"=w383:u8)  [unwired: 1 in, 2 out]
            n168 = Byte Array To String(unsigned byte array=w392) -> (string=w391:string)
            n169 = To Unsigned Long Integer(number=w384) -> (unsigned 32bit integer=w382:u32)
            n170 = To Unsigned Long Integer(number=w383) -> (unsigned 32bit integer=w381:u32)
            n171 = VISA Write(VISA resource name=w393, write buffer=w391, error in (no error)=w394) -> (VISA resource name out=w390:refnum<visa-resource-name>, error out=w389:errorcluster)  [unwired: 1 out]
            n172 = Multiply(x=w382, y=w381) -> (x*y=w380:u32)
            n173 = Add(x=w380, y=u32 2500) -> (x+y=w378:u32)
            n174 = flat-sequence {
              tunnel: w389 -> [w401]
              tunnel: [w401] -> w388
              tunnel: w378 -> [w400]
              frame #0 {
                n175 = Wait (ms)(milliseconds to wait=w400) -> ()  [unwired: 1 out]
              }
            }
            n176 = call "SDCP Request Start.vi"("error in (no error)"=w388, "COM Port"=w390) -> ("error out"=w374:errorcluster)  [unwired: 1 out]
            n177 = call "SDPC - Pause Transfer.vi"("error in (no error)"=w374, "Pause transfer"=FALSE) -> ("error out"=w373:errorcluster)  [unwired: 2 in, 1 out]
          }
          frame "RENC CLK" {
            n178 = call "SDPC - Pause Transfer.vi"("error in (no error)"=w419, "Pause transfer"=TRUE) -> ("error out"=w417:errorcluster)  [unwired: 2 in, 1 out]
            n179 = for {
              tunnel: w417 -> [w423]
              tunnel: [w422] -> w414
              tunnel: string[] ["RENC_CLK", "RENC_ACLK", "RENC_SW"] -> [w421] mode=indexing
              tunnel: dbl[] [0.0, 0.0, 0.0] -> [w420] mode=indexing
              n180 = call "SDCP - Write Parameter To Frame.vi"("error in (no error)"=w423, "Value"=w420, "Parameter Name"=w421) -> ("error out"=w422:errorcluster)  [unwired: 1 in, 1 out]
            }
            n181 = Unbundle By Name(w411) -> ("COM Port"=w410:refnum<vi>)
            n182 = property class="VISAName"(reference=w410) -> ("Value"=w408:refnum<visa-resource-name>)  [unwired: 1 in, 2 out]
            n183 = call "SDCP - Write Parameter To Frame.vi"("error in (no error)"=w414, "Value"=1.0, "Parameter Name"="RENC_CLK") -> ("error out"=w409:errorcluster, "Encoded message frame"=w407:u8[])  [unwired: 1 in]
            n184 = Byte Array To String(unsigned byte array=w407) -> (string=w406:string)
            n185 = VISA Write(VISA resource name=w408, write buffer=w406, error in (no error)=w409) -> (error out=w405:errorcluster)  [unwired: 2 out]
            n186 = call "SDPC - Pause Transfer.vi"("error in (no error)"=w405, "Pause transfer"=FALSE) -> ("error out"=w404:errorcluster)  [unwired: 2 in, 1 out]
          }
          frame "RENC ACLK" {
            n187 = call "SDPC - Pause Transfer.vi"("error in (no error)"=w441, "Pause transfer"=TRUE) -> ("error out"=w439:errorcluster)  [unwired: 2 in, 1 out]
            n188 = for {
              tunnel: w439 -> [w445]
              tunnel: [w444] -> w436
              tunnel: string[] ["RENC_CLK", "RENC_ACLK", "RENC_SW"] -> [w443] mode=indexing
              tunnel: dbl[] [0.0, 0.0, 0.0] -> [w442] mode=indexing
              n189 = call "SDCP - Write Parameter To Frame.vi"("error in (no error)"=w445, "Value"=w442, "Parameter Name"=w443) -> ("error out"=w444:errorcluster)  [unwired: 1 in, 1 out]
            }
            n190 = Unbundle By Name(w433) -> ("COM Port"=w432:refnum<vi>)
            n191 = property class="VISAName"(reference=w432) -> ("Value"=w430:refnum<visa-resource-name>)  [unwired: 1 in, 2 out]
            n192 = call "SDCP - Write Parameter To Frame.vi"("error in (no error)"=w436, "Value"=1.0, "Parameter Name"="RENC_ACLK") -> ("error out"=w431:errorcluster, "Encoded message frame"=w429:u8[])  [unwired: 1 in]
            n193 = Byte Array To String(unsigned byte array=w429) -> (string=w428:string)
            n194 = VISA Write(VISA resource name=w430, write buffer=w428, error in (no error)=w431) -> (error out=w427:errorcluster)  [unwired: 2 out]
            n195 = call "SDPC - Pause Transfer.vi"("error in (no error)"=w427, "Pause transfer"=FALSE) -> ("error out"=w426:errorcluster)  [unwired: 2 in, 1 out]
          }
          frame "RENC SW" {
            n196 = call "SDPC - Pause Transfer.vi"("error in (no error)"=w463, "Pause transfer"=TRUE) -> ("error out"=w461:errorcluster)  [unwired: 2 in, 1 out]
            n197 = for {
              tunnel: w461 -> [w467]
              tunnel: [w466] -> w458
              tunnel: string[] ["RENC_CLK", "RENC_ACLK", "RENC_SW"] -> [w465] mode=indexing
              tunnel: dbl[] [0.0, 0.0, 0.0] -> [w464] mode=indexing
              n198 = call "SDCP - Write Parameter To Frame.vi"("error in (no error)"=w467, "Value"=w464, "Parameter Name"=w465) -> ("error out"=w466:errorcluster)  [unwired: 1 in, 1 out]
            }
            n199 = Unbundle By Name(w455) -> ("COM Port"=w454:refnum<vi>)
            n200 = property class="VISAName"(reference=w454) -> ("Value"=w452:refnum<visa-resource-name>)  [unwired: 1 in, 2 out]
            n201 = call "SDCP - Write Parameter To Frame.vi"("error in (no error)"=w458, "Value"=1.0, "Parameter Name"="RENC_SW") -> ("error out"=w453:errorcluster, "Encoded message frame"=w451:u8[])  [unwired: 1 in]
            n202 = Byte Array To String(unsigned byte array=w451) -> (string=w450:string)
            n203 = VISA Write(VISA resource name=w452, write buffer=w450, error in (no error)=w453) -> (error out=w449:errorcluster)  [unwired: 2 out]
            n204 = call "SDPC - Pause Transfer.vi"("error in (no error)"=w449, "Pause transfer"=FALSE) -> ("error out"=w448:errorcluster)  [unwired: 2 in, 1 out]
          }
          frame Default {
          }
        }
      }
    }
    n205 = global read "Application Stop.vi" "Application Global Stop"() -> (w268:bool)
    n206 = And(x=w267, y=w268) -> (x .and. y?=w269:bool)
  }
  n207 = while {
    tunnel: w4 -> [w473]
    tunnel: w5 -> [w472]
    tunnel: [w470] -> _
    stop <- w474 stop-if-true
    # "Updation loop for parameters gathered from device"
    n208 = call "Gather data from device.vi"("error in (no error)"=w473, "Front Panel Object References"=w472) -> ("error out"=w471:errorcluster)  [unwired: 1 in]
    n209 = flat-sequence {
      tunnel: w471 -> [w476]
      tunnel: [w476] -> w470
      frame #0 {
        n210 = Wait (ms)(milliseconds to wait=u32 50) -> ()  [unwired: 1 out]
      }
    }
    n211 = global read "Application Stop.vi" "Application Global Stop"() -> (w474:bool)
  }
  n212 = while {
    tunnel: w4 -> [w484]
    tunnel: [w478] -> _
    stop <- w485 stop-if-true
    # "IMU sensor orientation rendering loop"
    n213 = local read "Pitch (degrees)"() -> (w481:dbl)
    n214 = local read "Roll (degrees)"() -> (w482:dbl)
    n215 = local read "Yaw (degrees)"() -> (w480:dbl)
    n216 = call "IMU orientation.vi"("Initialize ?"=FALSE, "error in (no error)"=w484, "Yaw"=w480, "Pitch"=w481, "Roll"=w482) -> ("error out"=w479:errorcluster, "3D Picture"=w477:refnum<vi>)  [unwired: 5 in]
    n217 = flat-sequence {
      tunnel: w479 -> [w487]
      tunnel: [w487] -> w478
      frame #0 {
        n218 = Wait (ms)(milliseconds to wait=u32 50) -> ()  [unwired: 1 out]
      }
    }
    n219 = local write "IMU orientation"(w477) -> ()
    n220 = global read "Application Stop.vi" "Application Global Stop"() -> (w485:bool)
  }
